vi "Read IPG Thermistor Temperature.vi"(8 "error in":errorcluster) -> (0 "error out":errorcluster, 1 "MICS Output":T1, 2 "Temperature (degC)":dbl)   [LabVIEW 2010]
uses:
  Zarlink Telemetry v9_0/Telemetry/Typedef Command List.ctl
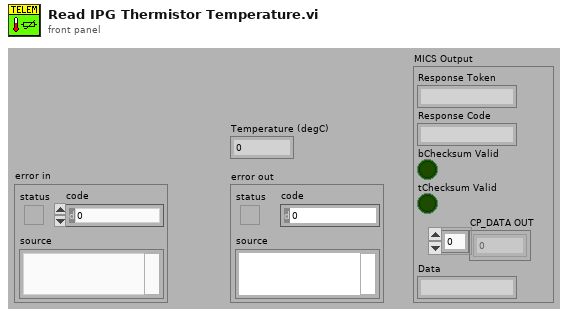
[diagram p1: front panel]
types:
  T1 = cluster{"Response Token":string, "Response Code":string, "bChecksum Valid":bool, "tChecksum Valid":bool, "CP_DATA OUT":u8[], "Data":string}
  T2 = typedef "Typedef Command List.ctl" = enum16{"Get xPG Status", "xPG Stimulation", "Select Program", "Increment Program Amplitude", "Decrement Program Amplitude", "Get PoP Constants", "Get PPC Constants", "Get Program Names", "Set Pulse Amplitude", "Increment Pulse Amplitude", "Decrement Pulse Amplitude", "Get Pulse Widths", "Set Pulse Widths", "Increment Pulse Width", "Decrement Pulse Width", "Get Program Frequency", "Set Program Frequency", "Increment Program Frequency", "Decrement Program Frequency", "<reserved 1>", "Charging Control", "Get xPG Identity", "Set xPG Identity", "Restore Program Defaults", "Get Program Definition", "Set Program Definition", "Get Program Constants", "Set Program Constants", "Get Configurable Device Parameters", "Set Configurable Device Parameters", "Get Pulse Constants", "Set Pulse Constants", "Get Lead Limits", "Set Lead Limits", "Get Channel Calibrations", "Set Channel Calibrations", "<reserved 2>", "<reserved 3>", "<reserved 4>", "<reserved 5>", "<reserved 6>", "<reserved 7>", "Get Stim Asic HV Calibrations", "Set Stim Asic HV Calibrations", "<reserved 8>", "<reserved 9>", "Get CP Data", "Set CP Data", "Clear Log", "Read Log", "Append Log", "Get Patient Program Runtime", "Set Patient Program Runtime", "Impedance Measurement", "Enter Storage Mode", "Echo Short", "Echo Long", "Get General Calibration", "Set General Calibration", "Get Trim List", "Set Trim List", "Get Counter", "Set Counter", "Get Test Stimulation", "Set Test Stimulation", "Get Titration Stimulation", "Set Titration Stimulation", "Get Ramp Time", "Set Ramp Time", "Get VBAT", "Set Software Description Block", "Get Software Description Block", "Write Memory", "Read Memory", "Reset xPG", "Erase Flash Block", "Write Vectors", "Read Vectors", "Diagnostic Data", "Set Background Impedance", "Get Background Impedence ", "Undefined"}
  T3 = cluster{"Command":T2, "Function":enum16{"Open Session", "Close Session", "Downlink Only", "Uplink Only", "Transceive (DN -> UP)"}, "MICS_ID":u32, "EXID":u32, "Use Local":bool, "Transceive Delay mS":dbl, "CP_DATA IN":u8[], "Parameters":string}
  T4 = enum16{"Open Session", "Close Session", "Downlink Only", "Uplink Only", "Transceive (DN -> UP)"}
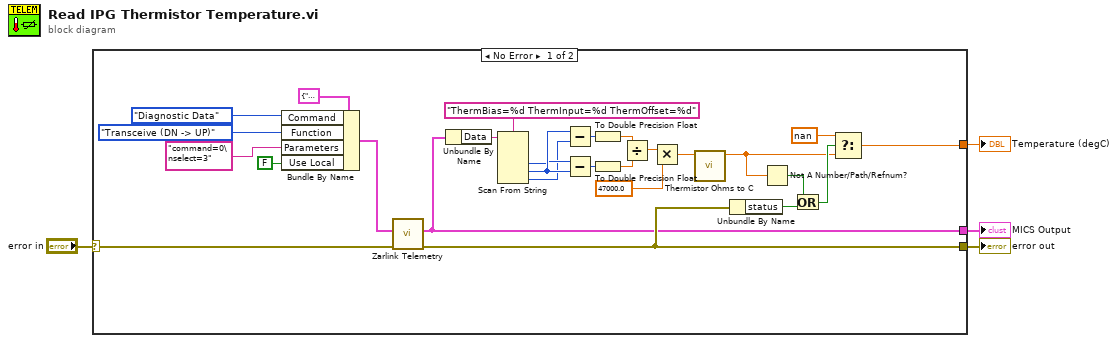
[diagram p0: block diagram]
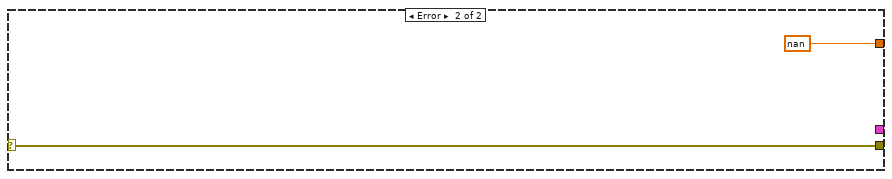
[diagram p2: hidden frame]
diagram:
  n1 = case shown="No Error" "error in" {
    selector: "error in" -> [w23 w33]
    tunnel: [w22 w33] -> w3
    tunnel: [w20 nan ("Temperature")] -> w2
    tunnel: [w18 _] -> w1
    frame No Error {
      n2 = Bundle By Name(cluster=T3 {"Command"=enum."Get xPG Status", "Function"=enum."Close Session", "MICS_ID"=0, "EXID"=16773121, "Use Local"=FALSE, "Transceive Delay mS"=100.0, "CP_DATA IN"=[], "Parameters"=""} ("Input"), "Command"=Typedef_Command_List."Diagnostic Data", "Function"=T4."Transceive (DN -> UP)", "Parameters"="command=0\nselect=3", "Use Local"=FALSE) -> (w28:T3)
      n3 = call "Zarlink Telemetry.vi"("error in (no error)"=w23, "Input"=w28) -> ("error out"=w22:errorcluster, "Output"=w18:T1)  [unwired: 7 in, 1 out]
      n4 = Unbundle By Name(w18) -> ("Data"=w6:string)
      n5 = Scan From String(format string="ThermBias=%d ThermInput=%d ThermOffset=%d", input string=w6) -> (output 1=w9:i32, output 2=w10:i32, output 3=w8:i32)  [unwired: 5 in, 3 out]
      n6 = Subtract(x=w10, y=w8) -> (x-y=w11:i32)
      n7 = Subtract(x=w9, y=w10) -> (x-y=w12:i32)
      n8 = To Double Precision Float(number=w11) -> (double precision float=w13:dbl)
      n9 = To Double Precision Float(number=w12) -> (double precision float=w14:dbl)
      n10 = Divide(x=w13, y=w14) -> (x/y=w15:dbl)
      n11 = Multiply(x=w15, y=47000.0) -> (x*y=w17:dbl)
      n12 = call "Thermistor Ohms to C.vi"("Thermistor R"=w17) -> ("Thermistor C"=w5:dbl)  [unwired: 10 in]
      n13 = Unbundle By Name(w22) -> ("status"=w30:bool)
      n14 = Not A Number/Path/Refnum?(number/path/refnum=w5) -> (NaN/Path/Refnum?=w31:bool)
      n15 = Or(x=w31, y=w30) -> (x .or. y?=w29:bool)
      n16 = Select(t=nan, s=w29, f=w5) -> (s? t:f=w20:dbl)
    }
    frame Error {
    }
  }
  "error out" <- w3
  "Temperature (degC)" <- w2
  "MICS Output" <- w1
